vi "Read_File_and_Set_Last_Modified.vi"(5 "file path":path) -> (0 "error out":errorcluster, 1 "string":string, 2 "file path Out":path)   [LabVIEW 2011]
uses:
  Globals/Trav_pos_global.vi
panel:
  out "substring":string
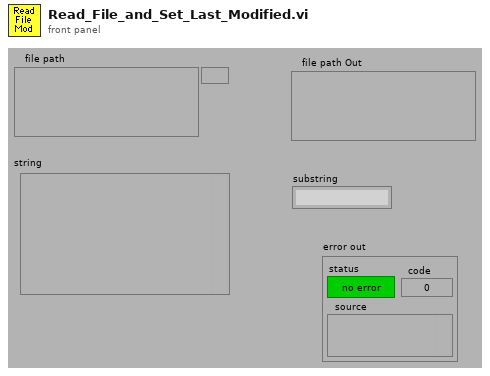
[diagram p1: front panel]
types:
  T1 = enum16{"deny read/write", "deny write-only", "deny none"}
  T2 = enum16{"open", "replace", "create", "open or create", "replace or create", "replace or create with confirmation"}
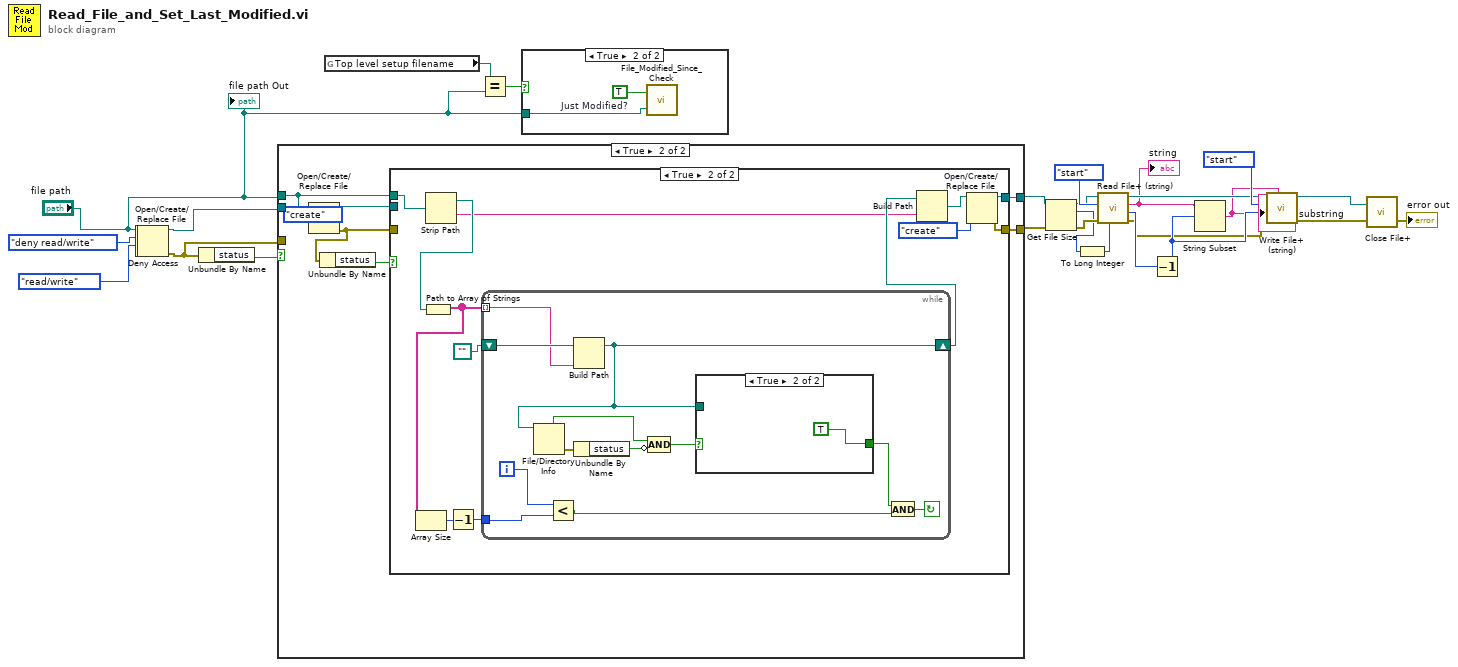
[diagram p0: block diagram]
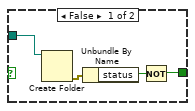
[diagram p5: hidden frame]
diagram:
  n1 = Open/Create/Replace File(file path (use dialog)="file path", access (0:read/write)=enum16{"read/write", "read-only", "write-only"}."read/write") -> (refnum out=w19:refnum<file>, error out=w20:errorcluster)  [unwired: 1 in, 4 out]
  n2 = Deny Access(4:w20, 6:T1."deny read/write" ("deny mode (2)"), 7:w19) -> (0:w22:errorcluster, 3:w25:refnum<file>)
  n3 = Unbundle By Name(w22) -> ("status"=w26:bool)
  n4 = case shown="True" w26 {
    tunnel: "file path" -> [_ w33]
    tunnel: w25 -> [w29 _]
    tunnel: [w29 w36] -> w10
    tunnel: [w28 w35] -> w8
    tunnel: w22 -> [w28 _]
    frame False {
    }
    frame True {
      n5 = Open/Create/Replace File(file path (use dialog)=w33, operation (0:open)=T2."create") -> (refnum out=w32:refnum<file>, error out=w31:errorcluster)  [unwired: 1 in, 4 out]
      n6 = Unbundle By Name(w31) -> ("status"=w34:bool)
      n7 = case shown="True" w34 {
        tunnel: w33 -> [_ w44]
        tunnel: [w38 w47] -> w36
        tunnel: [w37 w46] -> w35
        tunnel: w32 -> [w38 _]
        tunnel: w31 -> [w37 _]
        frame False {
        }
        frame True {
          n8 = Strip Path(path=w44) -> (stripped path=w43:path, name=w41:string)
          n9 = Path to Array of Strings(0:w43) -> (2:w49:string[])  [unwired: 1 out]
          n10 = Array Size(array=w49) -> (size(s)=w50:i32)
          n11 = Decrement(x=w50) -> (x-1=w48:i32)
          n12 = while {
            tunnel: w48 -> [w59]
            shift-left: path "" ("appended path") -> [w62]
            shift-right: [w55] -> w42
            tunnel: w49 -> [w61] mode=indexing
            i -> [w60]
            stop <- w57 continue-if-true
            n13 = Less?(x=w60, y=w59) -> (x < y?=w58:bool)
            n14 = Build Path(base path=w62, name or relative path=w61) -> (appended path=w55:path)
            n15 = File/Directory Info(path=w55) -> (directory=w52:bool, error out=w54:errorcluster)  [unwired: 1 in, 5 out]
            n16 = Unbundle By Name(w54) -> ("status"=w53:bool)
            n17 = Compound Arithmetic op=AND(w52, invert w53) -> (w51:bool)
            n18 = case shown="True" w51 {
              tunnel: w55 -> [w66 _]
              tunnel: [w63 TRUE] -> w56
              frame False {
                n19 = Create Folder(path (use dialog)=w66) -> (error out=w65:errorcluster)  [unwired: 1 in, 3 out]
                n20 = Unbundle By Name(w65) -> ("status"=w64:bool)
                n21 = Not(x=w64) -> (.not. x?=w63:bool)
              }
              frame True {
              }
            }
            n22 = And(x=w56, y=w58) -> (x .and. y?=w57:bool)
          }
          n23 = Build Path(base path=w42, name or relative path=w41) -> (appended path=w40:path)
          n24 = Open/Create/Replace File(file path (use dialog)=w40, operation (0:open)=T2."create") -> (refnum out=w47:refnum<file>, error out=w46:errorcluster)  [unwired: 1 in, 4 out]
        }
      }
    }
  }
  n25 = global read "Trav_pos_global.vi" "Top level setup filename"() -> (w2:path)
  n26 = Equal?(x=w2, y="file path") -> (x = y?=w3:bool)
  n27 = case shown="True" w3 {
    tunnel: "file path" -> [_ w68]
    frame False {
    }
    frame True {
      w69 = TRUE  # Just Modified?
      n28 = call "File_Modified_Since_Check.vi"("Pathname"=w68, "Just Modified?"=w69) -> ()  [unwired: 1 out]
    }
  }
  n29 = Get File Size(file=w10, error in=w8) -> (refnum out=w9:refnum<file>, size (in bytes)=w6:i64, 0:w7:errorcluster)
  n30 = To Long Integer(number=w6) -> (32bit integer=w5:i32)
  n31 = call <vilib>:"Read File+ (string).vi"("count"=w5, "error in (no error)"=w7, "pos mode (rel. to current:2)"=enum16{"start", "end", "current"}."start", "refnum"=w9) -> ("error out"=w13:errorcluster, "mark after read (bytes)"=w16:i32, "string"=w4:string, "dup refnum"=w12:refnum<file>)  [unwired: 1 in, 3 out]
  "string" <- w4
  n32 = Decrement(x=w16) -> (x-1=w14:i32)
  n33 = String Subset(string=w4, offset (0)=w14) -> (substring=w11:string)  [unwired: 1 in]
  "substring" <- w11
  n34 = call <vilib>:"Write File+ (string).vi"("string"=w11, "error in (no error)"=w13, "pos offset (bytes:0)"=w14, "pos mode (rel. to end:1)"=enum16{"start", "end", "current"}."start", "refnum"=w12) -> ("error out"=w24:errorcluster, "dup refnum"=w23:refnum<file>)  [unwired: 3 out]
  n35 = call <vilib>:"Close File+.vi"("error in (no error)"=w24, "refnum"=w23) -> ("error out"=→"error out":errorcluster)  [unwired: 5 out]
  "file path Out" <- "file path"
